vi "driveToHeading.vi"(10 "Speed (ft/sec)":dbl, 11 "Distance":dbl) -> ()   [LabVIEW 2011]
uses:
  <vilib>/Rock Robotics/WPI/DriverStation/DriverStationLCD/WPI_DriverStationLCDLCDLine.ctl
  drivetrain/drivetrain_drive_mode.ctl
  drivetrain/gear_shift_state.ctl
  drivetrain/drivetrain_drive_write_thread.ctl
  drivetrain/drivetrain_globals.vi
panel:
  out "Waveform Chart":dbl(graph)
  in  "gyro invert":bool=TRUE
  out "exit error":dbl
  in  "hdg gain":dbl=0.7
  in  "hdg target":dbl
  in  "gain":dbl=0.05
  in  "Bias":cluster{"Left":dbl, "Right":dbl}={"Left"=0.95, "Right"=1.0}
  in  "Max Delta Per Iteration":dbl=0.2
  in  "Overshoot":dbl=18.0
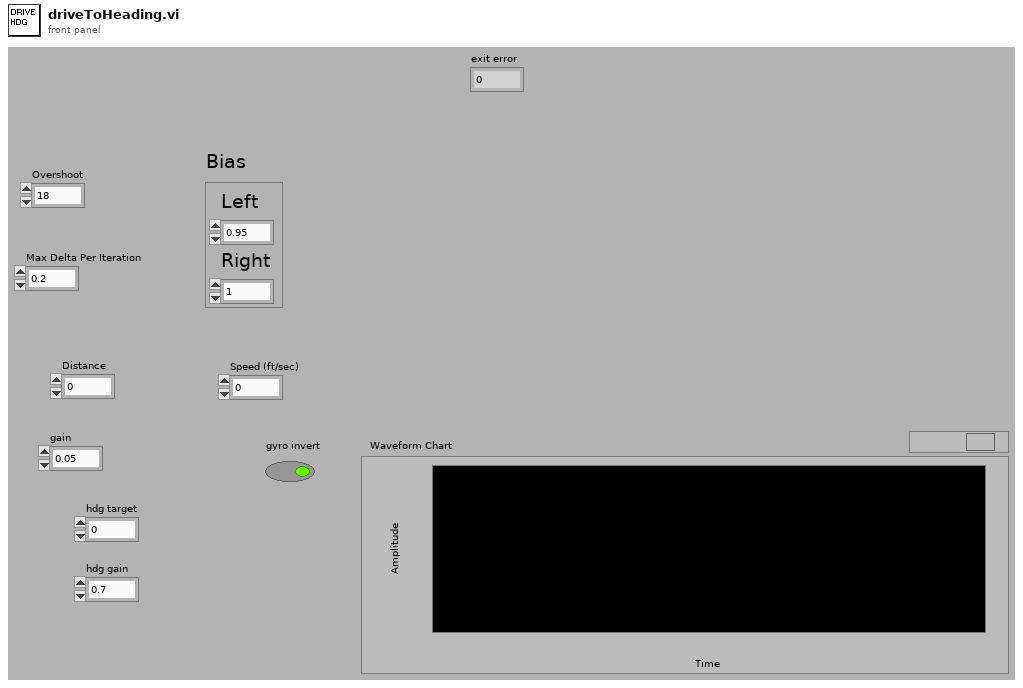
[diagram p1: front panel]
types:
  T1 = typedef "WPI_DriverStationLCDLCDLine.ctl" = enum16{"Main - Line 1", "User - Line 2", "User - Line 3", "User - Line 4", "User - Line 5", "User - Line 6"}
  T2 = typedef "drivetrain_drive_write_thread.ctl" = enum16{"Teleop", "Script Engine - Autonomous", "Script Engine - Sequence"}
  T3 = typedef "WPI_GyroDevRef.ctl" = cluster{"DevStatus":errorcluster, "Analog Module":T4, "Analog Channel":T5, "Offset":dbl, "Gain (VoltsPerDegree/Second)":dbl}
  T4 = typedef "FPGA_TypedefAnalogModule.ctl" = enum16{"Analog Module 1", "Analog Module 2"}
  T5 = typedef "FPGA_AIChannel.ctl" = enum8{"AI 1", "AI 2", "AI 3", "AI 4", "AI 5", "AI 6", "AI 7", "AI 8", "Invalid"}
  T6 = typedef "drivetrain_drive_mode.ctl" = enum16{"open loop", "closed loop"}
  T7 = typedef "gear_shift_state.ctl" = enum16{"low", "high"}
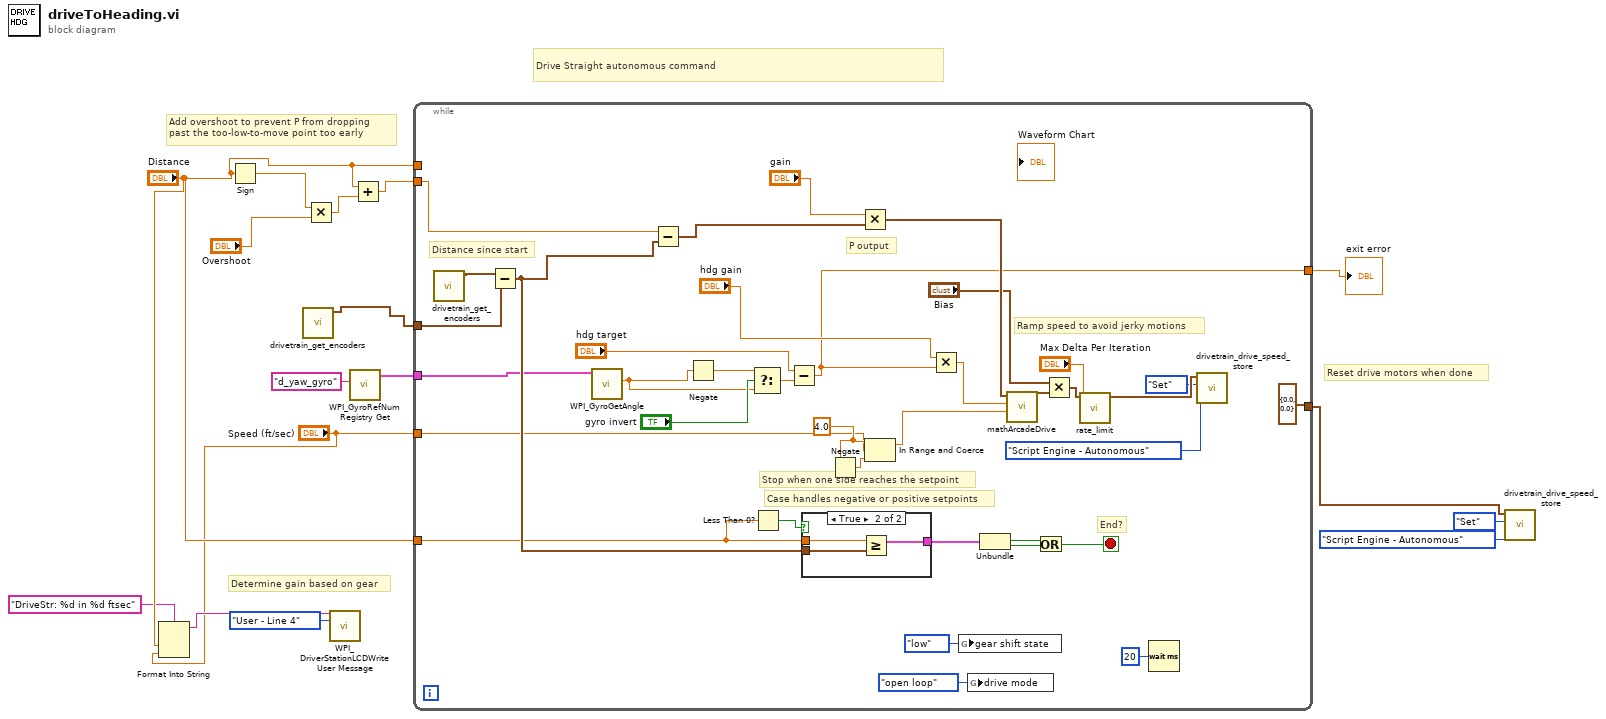
[diagram p0: block diagram]
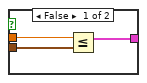
[diagram p2: hidden frame]
diagram:
  # "Determine gain based on gear"
  # "Drive Straight autonomous command"
  # "Reset drive motors when done"
  # "Add overshoot to prevent P from dropping\npast the too-low-to-move point too early"
  n1 = Format Into String(format string="DriveStr: %d in %d ftsec", "Distance", "Speed (ft/sec)") -> (resulting string=w5:string)  [unwired: 2 in, 1 out]
  n2 = Sign(1:"Distance") -> (0:w13:dbl)
  n3 = call "drivetrain_get_encoders.vi"() -> ("Distance (in)"=w10:cluster{"Left":dbl, "Right":dbl})  [unwired: 9 in, 2 out]
  n4 = Multiply(x=w13, y="Overshoot") -> (x*y=w15:dbl)
  n5 = call <vilib>:"WPI_DriverStationLCDWrite User Message.vi"("line text"=w5, "line"=WPI_DriverStationLCDLCDLine."User - Line 4") -> ()  [unwired: 13 in, 1 out]
  n6 = call <vilib>:"WPI_GyroRefNum Registry Get.vi"("refnum name"="d_yaw_gyro") -> ("GyroDevRef"=w11:T3)  [unwired: 1 in, 9 out]
  n7 = Add(x="Distance", y=w15) -> (x+y=w16:dbl)
  n8 = while {
    tunnel: "Speed (ft/sec)" -> [w21]
    tunnel: w10 -> [w53]
    tunnel: w16 -> [w45]
    tunnel: [cluster{"Left":dbl, "Right":dbl} {"Left"=0.0, "Right"=0.0} ("Drive")] -> w7
    tunnel: "Distance" -> [w34]
    tunnel: w11 -> [w33]
    tunnel: [w22] -> w6
    tunnel: "Distance" -> [_]
    stop <- w49 stop-if-true
    w41 = 4.0
    # "Case handles negative or positive setpoints"
    # "End?"
    # "Ramp speed to avoid jerky motions"
    # "P output"
    # "Stop when one side reaches the setpoint"
    # "Distance since start"
    n9 = call "drivetrain_get_encoders.vi"() -> ("Distance (in)"=w31:cluster{"Left":dbl, "Right":dbl})  [unwired: 9 in, 2 out]
    n10 = Subtract(x=w31, y=w53) -> (x-y=w38:cluster{"Left":dbl, "Right":dbl})
    n11 = call <vilib>:"WPI_GyroGetAngle.vi"("GyroDevRef"=w33) -> ("Angle"=w17:dbl)  [unwired: 1 in, 9 out]
    n12 = Subtract(x=w45, y=w38) -> (x-y=w46:cluster{"Left":dbl, "Right":dbl})
    n13 = Negate(x=w17) -> (-x=w18:dbl)
    n14 = Select(t=w18, s="gyro invert", f=w17) -> (s? t:f=w19:dbl)
    n15 = Less Than 0?(x=w34) -> (x < 0?=w44:bool)
    n16 = Subtract(x="hdg target", y=w19) -> (x-y=w22:dbl)
    n17 = case shown="True" w44 {
      tunnel: w34 -> [w56 w59]
      tunnel: w38 -> [w55 w58]
      tunnel: [w54 w57] -> w52
      frame False {
        n18 = Less Or Equal?(x=w56, y=w55) -> (x <= y?=w54:cluster{"Left":bool, "Right":bool})
      }
      frame True {
        n19 = Greater Or Equal?(x=w59, y=w58) -> (x >= y?=w57:cluster{"Left":bool, "Right":bool})
      }
    }
    n20 = Negate(x=w41) -> (-x=w42:dbl)
    n21 = Multiply(x="gain", y=w46) -> (x*y=w39:cluster{"Left":dbl, "Right":dbl})
    n22 = In Range and Coerce(upper limit=w41, x=w21, lower limit=w42) -> (coerced(x)=w40:dbl)  [unwired: 1 out]
    n23 = Multiply(x="hdg gain", y=w22) -> (x*y=w32:dbl)
    n24 = global write "drivetrain_globals.vi" "gear shift state"(gear_shift_state."low" ("gear shift state")) -> ()
    n25 = global write "drivetrain_globals.vi" "drive mode"(drivetrain_drive_mode."open loop" ("drive mode")) -> ()
    n26 = Unbundle(w52) -> ("Left"=w51:bool, "Right"=w50:bool)
    n27 = call "mathArcadeDrive.vi"("Range"=w40, "Wheel"=w32, "Throttle"=w39) -> ("Drive"=w37:cluster{"Left":dbl, "Right":dbl})  [unwired: 8 in]
    n28 = Or(x=w51, y=w50) -> (x .or. y?=w49:bool)
    n29 = Multiply(x="Bias", y=w37) -> (x*y=w36:cluster{"Left":dbl, "Right":dbl})
    n30 = call "rate_limit.vi"("Max Delta Per Iteration"="Max Delta Per Iteration", "Drive"=w36) -> ("Output"=w30:cluster{"Left":dbl, "Right":dbl})  [unwired: 9 in]
    n31 = Wait (ms)(milliseconds to wait=u32 20) -> ()  [unwired: 1 out]
    n32 = call "drivetrain_drive_speed_store.vi"("Write Thread"=drivetrain_drive_write_thread."Script Engine - Autonomous", "data_store_mode"=enum16{"Set", "Get"}."Set", "drive data"=w30) -> ()  [unwired: 8 in, 1 out]
  }
  "exit error" <- w6
  n33 = call "drivetrain_drive_speed_store.vi"("Write Thread"=drivetrain_drive_write_thread."Script Engine - Autonomous", "data_store_mode"=enum16{"Set", "Get"}."Set", "drive data"=w7) -> ()  [unwired: 8 in, 1 out]
